vi "New Test.vi"(5 "timeout ms (-1)":i32=-1, 6 "Station":T1(ring), 7 "Socket":i32, 8 "error in (no error)":errorcluster, 11 "Test":string) -> (0 "error out":errorcluster)   [LabVIEW 2019, in "Unit Test Engine Tools.lvlib"]
uses:
  Unit Test Engine Tools.lvlib
  LVUT Global 1.vi
  <resource>/objmgr/ni.dex.rc
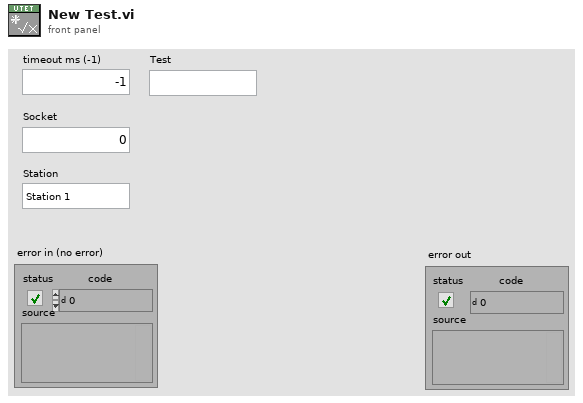
[diagram p1: front panel]
types:
  T1 = enum16{"Station 1", "Station 2", "Station 3", "Station 4"}
  T2 = cluster{"Socket":i32, "StepName":string, "Sequence Path":string[]}
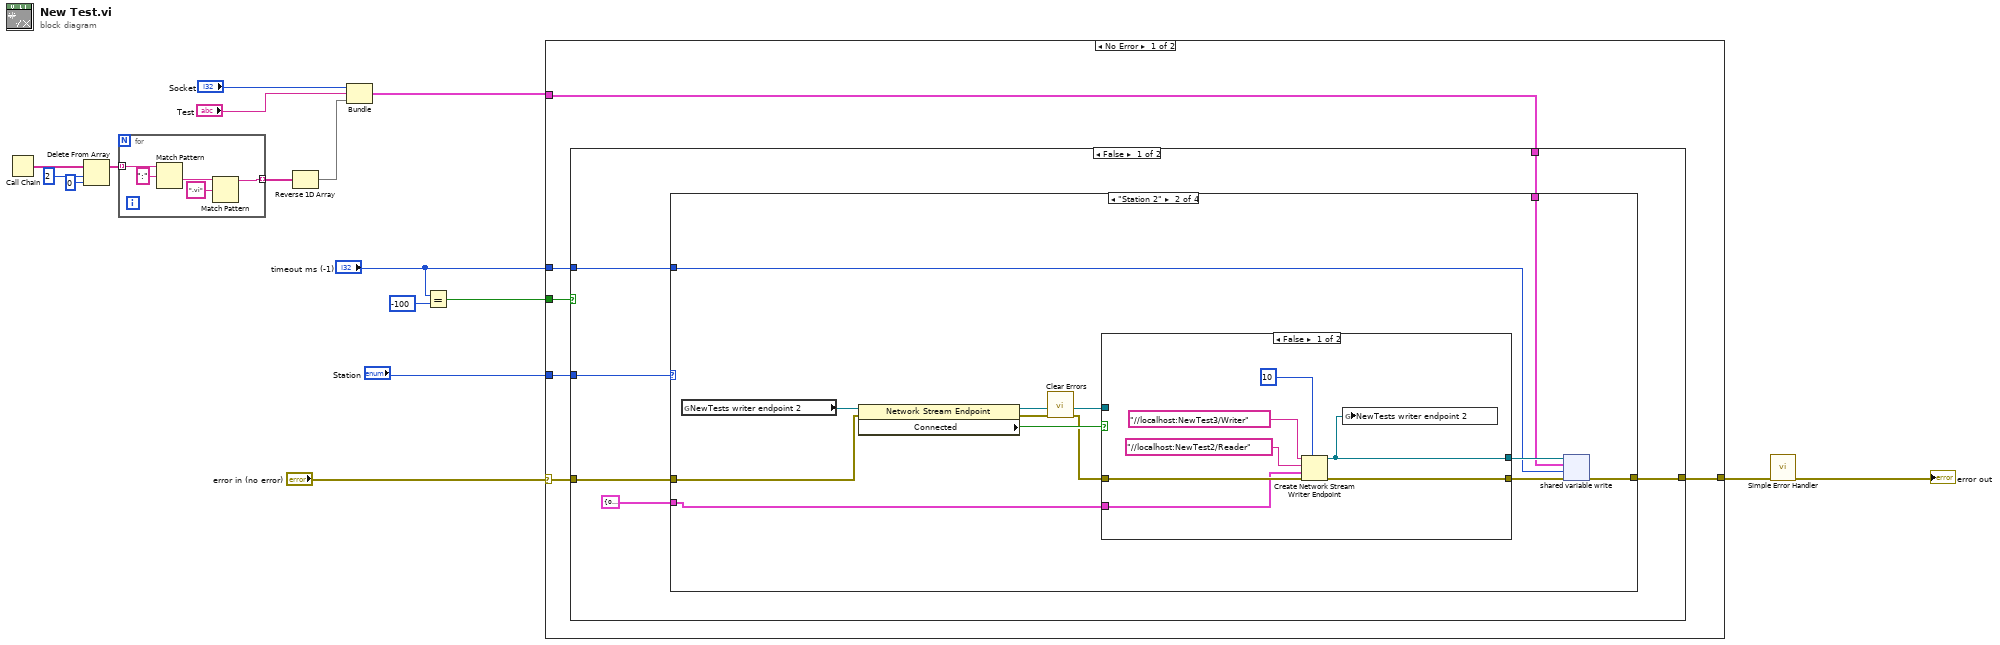
[diagram p0: block diagram]
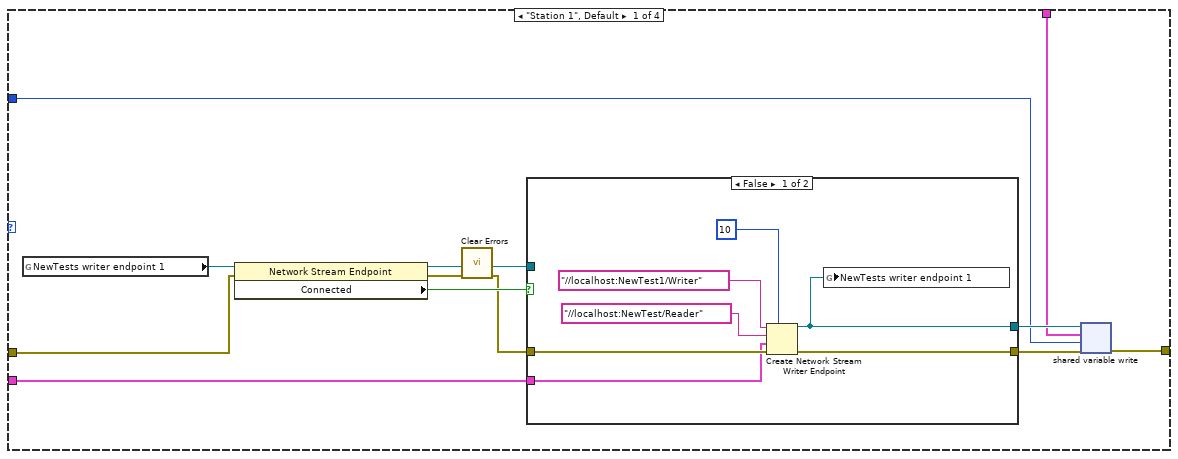
[diagram p2: hidden frame]
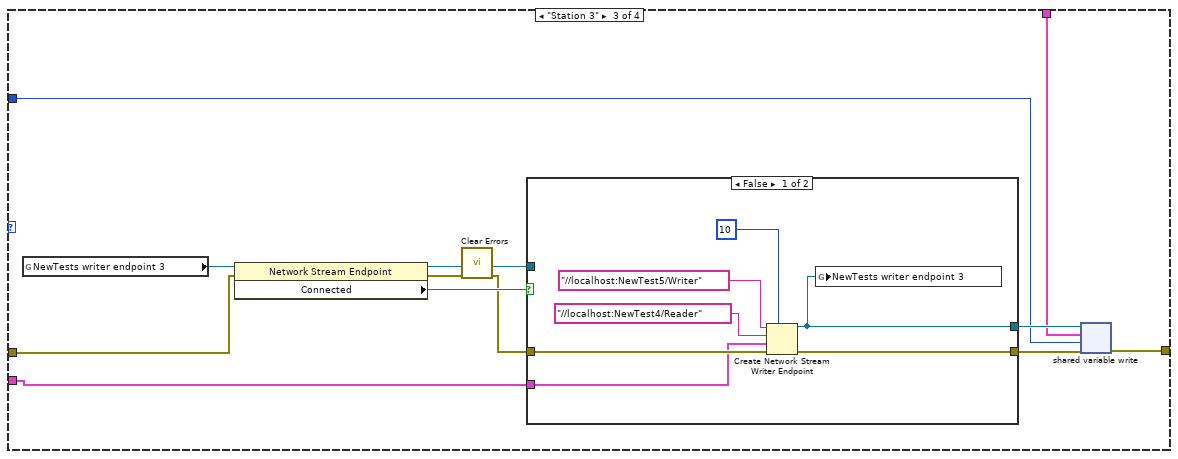
[diagram p5: hidden frame]
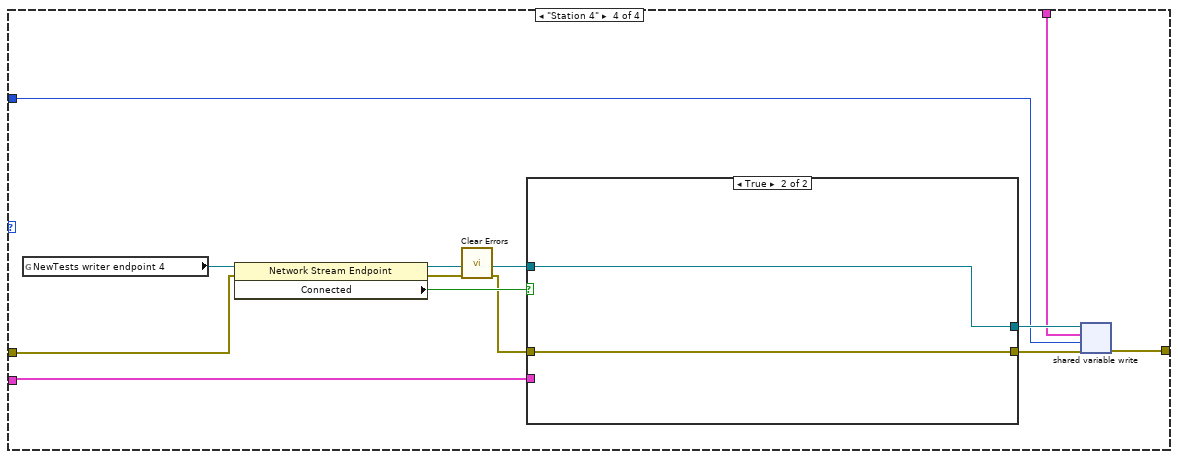
[diagram p7: hidden frame]
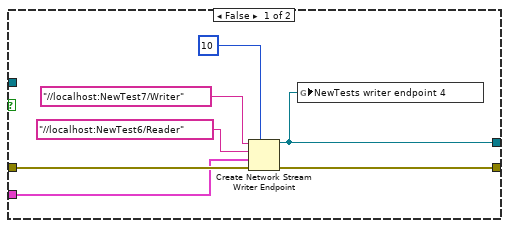
[diagram p8: hidden frame]
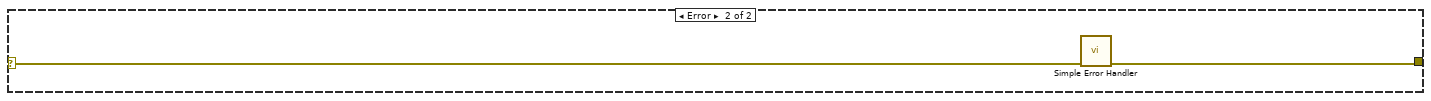
[diagram p10: hidden frame]
diagram:
  n1 = Call Chain() -> (call chain=w6:string[])
  n2 = Delete From Array(array=w6, length=2, index=0) -> (array with subset deleted=w3:string[])  [unwired: 1 out]
  n3 = for {
    tunnel: w3 -> [w21] mode=indexing
    tunnel: [w18] -> w2 mode=indexing
    n4 = Match Pattern(string=w21, regular expression=":") -> (after substring=w19:string)  [unwired: 1 in, 3 out]
    n5 = Match Pattern(string=w19, regular expression=".vi") -> (before substring=w18:string)  [unwired: 1 in, 3 out]
  }
  n6 = Reverse 1D Array(array=w2) -> (reversed array=w1:string[])
  n7 = Bundle("Socket"="Socket", "Test"="Test", w1) -> (w14:cluster{"Socket":i32, "Test":string, string[]})  [unwired: 1 in]
  n8 = Equal?(x="timeout ms (-1)", y=-100) -> (x = y?=w7:bool)
  n9 = case shown="No Error" "error in (no error)" {
    selector: "error in (no error)" -> [w24 w120]
    tunnel: "timeout ms (-1)" -> [w27 _]
    tunnel: w14 -> [w26 _]
    tunnel: [w25 w119] -> w13
    tunnel: "Station" -> [w23 _]
    tunnel: w7 -> [w22 _]
    frame No Error {
      n10 = case shown="False" w22 {
        tunnel: w27 -> [w33 _]
        tunnel: w26 -> [w32 _]
        tunnel: [w31 w118] -> w25
        tunnel: w24 -> [w30 w118]
        tunnel: w23 -> [w29 _]
        frame False {
          n11 = case shown="\"Station 2\"" w29 {
            tunnel: w33 -> [w43 w64 w85 w106]
            tunnel: w32 -> [w42 w63 w84 w105]
            tunnel: [w37 w58 w79 w100] -> w31
            tunnel: w30 -> [w36 w57 w78 w99]
            tunnel: T2 {"Socket"=0, "StepName"="", "Sequence Path"=[]} -> [w34 w55 w76 w97]
            frame "Station 1", Default {
              n12 = global read "LVUT Global 1.vi" "NewTests writer endpoint 1"() -> (w41:refnum<k21>)
              n13 = property class="Network Stream Endpoint"(reference=w41, error in=w36) -> (reference out=w38:refnum<k21>, error out=w40:errorcluster, "Connected"=w39:bool)
              n14 = call <vilib>:"Clear Errors.vi"("error in (no error)"=w40) -> ("error out"=w35:errorcluster)  [unwired: 5 in, 1 out]
              n15 = case shown="False" w39 {
                tunnel: [w46 w54] -> w45
                tunnel: [w50 w53] -> w44
                tunnel: w35 -> [w48 w53]
                tunnel: w38 -> [_ w54]
                tunnel: w34 -> [w47 _]
                frame False {
                  n16 = Create Network Stream Writer Endpoint(7:10 ("writer buffer size"), 8:w48, 9:w47, 10:"//localhost:NewTest/Reader" ("reader name"), 11:"//localhost:NewTest1/Writer" ("reader name")) -> (0:w50:errorcluster, 3:w46:refnum<k21>)  [unwired: 2 in]
                  n17 = global write "LVUT Global 1.vi" "NewTests writer endpoint 1"(w46) -> ()
                }
                frame True {
                }
              }
              n18 = shared-variable-write(w45, w44, w42, w43) -> (w37:errorcluster)  [unwired: 2 out]
            }
            frame "Station 2" {
              n19 = global read "LVUT Global 1.vi" "NewTests writer endpoint 2"() -> (w62:refnum<k21>)
              n20 = property class="Network Stream Endpoint"(reference=w62, error in=w57) -> (reference out=w59:refnum<k21>, error out=w61:errorcluster, "Connected"=w60:bool)
              n21 = call <vilib>:"Clear Errors.vi"("error in (no error)"=w61) -> ("error out"=w56:errorcluster)  [unwired: 5 in, 1 out]
              n22 = case shown="False" w60 {
                tunnel: [w68 w75] -> w66
                tunnel: [w71 w74] -> w65
                tunnel: w56 -> [w69 w74]
                tunnel: w59 -> [_ w75]
                tunnel: w55 -> [w67 _]
                frame False {
                  n23 = Create Network Stream Writer Endpoint(7:10 ("writer buffer size"), 8:w69, 9:w67, 10:"//localhost:NewTest2/Reader" ("reader name"), 11:"//localhost:NewTest3/Writer" ("reader name")) -> (0:w71:errorcluster, 3:w68:refnum<k21>)  [unwired: 2 in]
                  n24 = global write "LVUT Global 1.vi" "NewTests writer endpoint 2"(w68) -> ()
                }
                frame True {
                }
              }
              n25 = shared-variable-write(w66, w65, w63, w64) -> (w58:errorcluster)  [unwired: 2 out]
            }
            frame "Station 3" {
              n26 = global read "LVUT Global 1.vi" "NewTests writer endpoint 3"() -> (w83:refnum<k21>)
              n27 = property class="Network Stream Endpoint"(reference=w83, error in=w78) -> (reference out=w80:refnum<k21>, error out=w82:errorcluster, "Connected"=w81:bool)
              n28 = call <vilib>:"Clear Errors.vi"("error in (no error)"=w82) -> ("error out"=w77:errorcluster)  [unwired: 5 in, 1 out]
              n29 = case shown="False" w81 {
                tunnel: [w89 w96] -> w87
                tunnel: [w92 w95] -> w86
                tunnel: w77 -> [w90 w95]
                tunnel: w80 -> [_ w96]
                tunnel: w76 -> [w88 _]
                frame False {
                  n30 = Create Network Stream Writer Endpoint(7:10 ("writer buffer size"), 8:w90, 9:w88, 10:"//localhost:NewTest4/Reader" ("reader name"), 11:"//localhost:NewTest5/Writer" ("reader name")) -> (0:w92:errorcluster, 3:w89:refnum<k21>)  [unwired: 2 in]
                  n31 = global write "LVUT Global 1.vi" "NewTests writer endpoint 3"(w89) -> ()
                }
                frame True {
                }
              }
              n32 = shared-variable-write(w87, w86, w84, w85) -> (w79:errorcluster)  [unwired: 2 out]
            }
            frame "Station 4" {
              n33 = global read "LVUT Global 1.vi" "NewTests writer endpoint 4"() -> (w104:refnum<k21>)
              n34 = property class="Network Stream Endpoint"(reference=w104, error in=w99) -> (reference out=w101:refnum<k21>, error out=w103:errorcluster, "Connected"=w102:bool)
              n35 = call <vilib>:"Clear Errors.vi"("error in (no error)"=w103) -> ("error out"=w98:errorcluster)  [unwired: 5 in, 1 out]
              n36 = case shown="True" w102 {
                tunnel: [w110 w117] -> w108
                tunnel: [w113 w116] -> w107
                tunnel: w98 -> [w111 w116]
                tunnel: w101 -> [_ w117]
                tunnel: w97 -> [w109 _]
                frame False {
                  n37 = Create Network Stream Writer Endpoint(7:10 ("writer buffer size"), 8:w111, 9:w109, 10:"//localhost:NewTest6/Reader" ("reader name"), 11:"//localhost:NewTest7/Writer" ("reader name")) -> (0:w113:errorcluster, 3:w110:refnum<k21>)  [unwired: 2 in]
                  n38 = global write "LVUT Global 1.vi" "NewTests writer endpoint 4"(w110) -> ()
                }
                frame True {
                }
              }
              n39 = shared-variable-write(w108, w107, w105, w106) -> (w100:errorcluster)  [unwired: 2 out]
            }
          }
        }
        frame True {
        }
      }
    }
    frame Error {
      n40 = call <vilib>:"Simple Error Handler.vi"("error in (no error)"=w120) -> ("error out"=w119:errorcluster)  [unwired: 4 in, 4 out]
    }
  }
  n41 = call <vilib>:"Simple Error Handler.vi"("error in (no error)"=w13) -> ("error out"=→"error out":errorcluster)  [unwired: 4 in, 4 out]
